vi "Loader_SPI.vi"(4 "SPI_Mode":T1, 6 "Pattern Name":string, 7 "PinMap":path, 8 "error in (no error)":errorcluster, 9 "Timeset between frms":u32=50, 10 "SPI Frame Array":refnum<class "SPI_Frame_Root.lvclass">[](array[class]), 11 "DigiPattern_Generator.lvclass":refnum<class "DigiPattern_Generator.lvclass">) -> (0 "error out":errorcluster, 3 "DigiPattern_Generator.lvclass out":refnum<class "DigiPattern_Generator.lvclass">)   [LabVIEW 2018, in "DigiPattern_Generator.lvclass"]
uses:
  DigiPattern_Generator.lvclass
  SPI/SPI Frame Root/SPI_Frame_Root.lvclass
  SPI/Config Read SPI/SPI_Mode.ctl
  DigiPattern_Generator.lvclass/DigiPattern_Generator.ctl
  SPI/Config Read SPI/Config_Read_SPI.lvclass
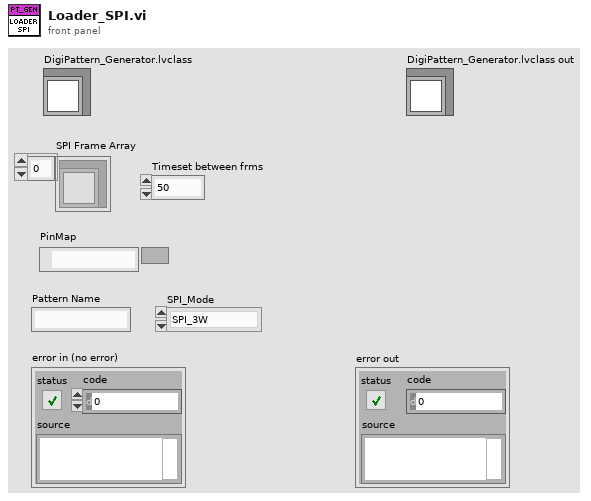
[diagram p1: front panel]
types:
  T1 = typedef "Config_Read_SPI.lvclass/SPI_Mode.ctl" = enum16{"SPI_3W", "SPI_4W"}
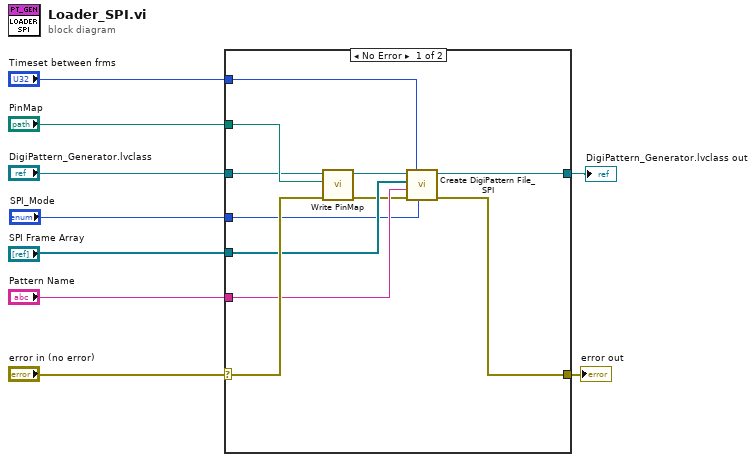
[diagram p0: block diagram]
diagram:
  n1 = case shown="No Error" "error in (no error)" {
    selector: "error in (no error)" -> [w18 w21]
    tunnel: "DigiPattern_Generator.lvclass" -> [w19 w22]
    tunnel: "PinMap" -> [w20 _]
    tunnel: "SPI Frame Array" -> [w14 _]
    tunnel: "Pattern Name" -> [w13 _]
    tunnel: [w15 w22] -> w5
    tunnel: [w11 w21] -> w4
    tunnel: "Timeset between frms" -> [w17 _]
    tunnel: "SPI_Mode" -> [w10 _]
    frame No Error {
      n2 = call "Write PinMap.vi"("error in (no error)"=w18, "PinMap"=w20, "BML_DigiPattern_Generator in"=w19) -> ("error out"=w12:errorcluster, "BML_DigiPattern_Generator out"=w16:refnum<class "DigiPattern_Generator.lvclass">)  [unwired: 7 in]
      n3 = call "Create DigiPattern File_SPI.vi"("SPI_Mode"=w10, "Timeset between frms"=w17, "error in (no error)"=w12, "Pattern Name"=w13, "SPI FRM"=w14, "DigiPattern_Generator.lvclass"=w16) -> ("error out"=w11:errorcluster, "DigiPattern_Generator.lvclass out"=w15:refnum<class "DigiPattern_Generator.lvclass">)  [unwired: 4 in]
    }
    frame Error {
    }
  }
  "DigiPattern_Generator.lvclass out" <- w5
  "error out" <- w4
